vi "test Process Records.vi"(8 "error in":errorcluster, 11 "TestCase in":refnum<class "Engine.lvclass">) -> (0 "error out":errorcluster, 3 "TestCase out":refnum<class "Engine.lvclass">)   [LabVIEW 2020, in "Engine.lvclass"]
uses:
  Engine.lvclass
  Shared/RT Hardware Channel Settings.ctl
  Shared/RT Label Settings.ctl
  Shared/Label.ctl
  Shared/RT Parameters.ctl
  Shared/Parameter Definition.ctl
  <vilib>/NI/NI VeriStand Encoding and Decoding/Encoding.ctl
  <vilib>/NI VeriStand/Custom Device API/Custom Device Item Ref.ctl
  Shared/Transfer Type.ctl
  <vilib>/NI VeriStand/Custom Device API/Data Reference.ctl
  Shared/Map of Identifiers to Indexes.ctl
  <vilib>/addons/_JKI Toolkits/VI Tester/TestCase.llb/TestCase.lvclass
  <vilib>/NI VeriStand/Custom Device API/Custom Device API.lvlib
  <vilib>/NI/NI VeriStand Encoding and Decoding/Encoding and Decoding.lvlib
  Engine/Custom Device/Custom Device.lvlib
  Hardware API/AIM ARINC 429 Hardware API.lvlib
  C:/Program Files (x86)/National Instruments/LabVIEW 2020/vi.lib/addons/_JKI Toolkits/VI Tester/TestCase.llb/TestCase.lvclass
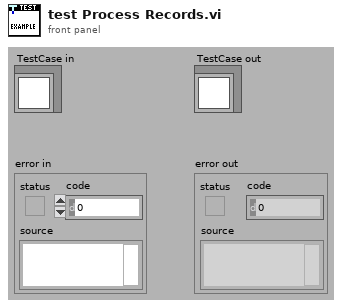
[diagram p1: front panel]
types:
  T1 = cluster{"type":u16, "count":u16, "timestamp":u32, "msgact":u16, "decgap":u16, "data":u32, "timestamph":u32}[]
  T2 = typedef "RT Hardware Channel Settings.ctl" = cluster{"channel #":u16, "channel handle":u64, "labels settings for RT":T3[]}
  T3 = typedef "RT Label Settings.ctl" = cluster{"Name":string, "xmlName":string, "label":T4, "transfer period":u32, "SDI_Enabled":bool, "SDI":u8, "parameter driver data":T5, "transfer type":T9, "has timestamp?":bool, "Label Disable/Trigger Channel Reference":T8, "Message Handle":u64, "Initialized?":bool, "Word Initial Raw Value":u32, "Label Timestamp Channel Data Reference":T10, "disabled":bool}
  T4 = typedef "Label.ctl" = u8
  T5 = typedef "RT Parameters.ctl" = cluster{"parameter definitions":T6[], "Tx parameter refs":T8[]}
  T6 = typedef "Parameter Definition.ctl" = cluster{"start index":i32, "size":i32, "encoding":T7, "signed":bool, "scale multiplier":dbl, "scale offset":dbl}
  T7 = typedef "Encoding and Decoding.lvlib/Encoding.ctl" = enum16{"BNR", "BCD", "Discrete"}
  T8 = typedef "Custom Device API.lvlib/Custom Device Item Ref.ctl" = u64
  T9 = typedef "Transfer Type.ctl" = enum16{"Scheduled", "Acyclic", "Block", "Strobe"}
  T10 = typedef "Custom Device API.lvlib/Data Reference.ctl" = i32
  T11 = typedef "Map of Identifiers to Indexes.ctl" = map{cluster{"Port":u8, "Label":u8, "SDI":u8}, cluster{"channel index":i32, "label index":i32, "start index":i32, "parameters":i32, "timestamp index":i32}}
  T12 = map{cluster{"hardware channel":u8, "label":u8, "SDI":u8}, cluster{"data word":u32, "time stamp":dbl}}
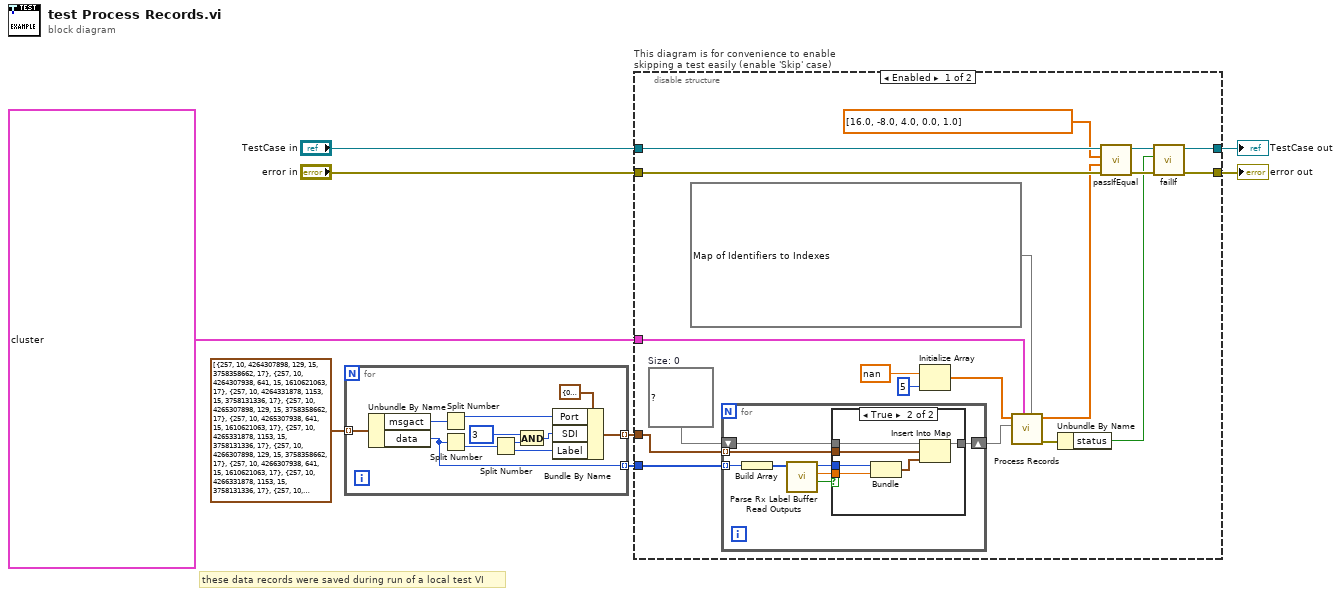
[diagram p0: block diagram]
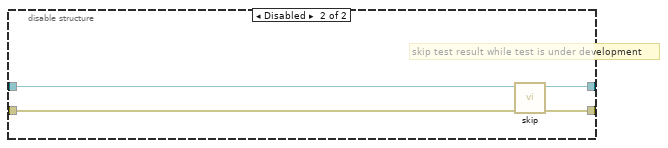
[diagram p3: hidden frame]
diagram:
  # "these data records were saved during run of a local test VI"
  n1 = for {
    tunnel: T1 [{"type"=257, "count"=10, "timestamp"=4264307898, "msgact"=129, "decgap"=15, "data"=3758358662, "timestamph"=17}, {"type"=257, "count"=10, "timestamp"=4264307938, "msgact"=641, "decgap"=15, "data"=1610621063, "timestamph"=17}, {"type"=257, "count"=10, "timestamp"=4264331878, "msgact"=1153, "decgap"=15, "data"=3758131336, "timestamph"=17}, {"type"=257, "count"=10, "timestamp"=4265307898, "msgact"=129, "decgap"=15, "data"=3758358662, "timestamph"=17}, {"type"=257, "count"=10, "timestamp"=4265307938, "msgact"=641, "decgap"=15, "data"=1610621063, "timestamph"=17}, {"type"=257, "count"=10, "timestamp"=4265331878, "msgact"=1153, "decgap"=15, "data"=3758131336, "timestamph"=17}, {"type"=257, "count"=10, "timestamp"=4266307898, "msgact"=129, "decgap"=15, "data"=3758358662, "timestamph"=17}, {"type"=257, "count"=10, "timestamp"=4266307938, "msgact"=641, "decgap"=15, "data"=1610621063, "timestamph"=17}, {"type"=257, "count"=10, "timestamp"=4266331878, "msgact"=1153, "decgap"=15, "data"=3758131336, "timestamph"=17}, {"type"=257, "count"=10, "timestamp"=4267307898, "msgact"=129, "decgap"=15, "data"=3758358662, "timestamph"=17}, {"type"=257, "count"=10, "timestamp"=4267307938, "msgact"=641, "decgap"=15, "data"=1610621063, "timestamph"=17}, {"type"=257, "count"=10, "timestamp"=4267331858, "msgact"=1153, "decgap"=15, "data"=3758131336, "timestamph"=17}, {"type"=257, "count"=10, "timestamp"=4268307898, "msgact"=129, "decgap"=15, "data"=3758358662, "timestamph"=17}, {"type"=257, "count"=10, "timestamp"=4268307938, "msgact"=641, "decgap"=15, "data"=1610621063, "timestamph"=17}, {"type"=257, "count"=10, "timestamp"=4268331858, "msgact"=1153, "decgap"=15, "data"=3758131336, "timestamph"=17}, {"type"=257, "count"=10, "timestamp"=4269307898, "msgact"=129, "decgap"=15, "data"=3758358662, "timestamph"=17}, {"type"=257, "count"=10, "timestamp"=4269307938, "msgact"=641, "decgap"=15, "data"=1610621063, "timestamph"=17}, {"type"=257, "count"=10, "timestamp"=4269331858, "msgact"=1153, "decgap"=15, "data"=3758131336, "timestamph"=17}, {"type"=257, "count"=10, "timestamp"=4270307898, "msgact"=129, "decgap"=15, "data"=3758358662, "timestamph"=17}, {"type"=257, "count"=10, "timestamp"=4270307938, "msgact"=641, "decgap"=15, "data"=1610621063, "timestamph"=17}, {"type"=257, "count"=10, "timestamp"=4270331878, "msgact"=1153, "decgap"=15, "data"=3758131336, "timestamph"=17}, {"type"=257, "count"=10, "timestamp"=4271307898, "msgact"=129, "decgap"=15, "data"=3758358662, "timestamph"=17}, {"type"=257, "count"=10, "timestamp"=4271307938, "msgact"=641, "decgap"=15, "data"=1610621063, "timestamph"=17}, {"type"=257, "count"=10, "timestamp"=4271331858, "msgact"=1153, "decgap"=15, "data"=3758131336, "timestamph"=17}, {"type"=257, "count"=10, "timestamp"=4272307898, "msgact"=129, "decgap"=15, "data"=3758358662, "timestamph"=17}, {"type"=257, "count"=10, "timestamp"=4272307938, "msgact"=641, "decgap"=15, "data"=1610621063, "timestamph"=17}, {"type"=257, "count"=10, "timestamp"=4272331858, "msgact"=1153, "decgap"=15, "data"=3758131336, "timestamph"=17}, {"type"=257, "count"=10, "timestamp"=4273307898, "msgact"=129, "decgap"=15, "data"=3758358662, "timestamph"=17}, {"type"=257, "count"=10, "timestamp"=4273307938, "msgact"=641, "decgap"=15, "data"=1610621063, "timestamph"=17}, {"type"=257, "count"=10, "timestamp"=4273331878, "msgact"=1153, "decgap"=15, "data"=3758131336, "timestamph"=17}, {"type"=257, "count"=10, "timestamp"=4274307898, "msgact"=129, "decgap"=15, "data"=3758358662, "timestamph"=17}, {"type"=257, "count"=10, "timestamp"=4274307938, "msgact"=641, "decgap"=15, "data"=1610621063, "timestamph"=17}, {"type"=257, "count"=10, "timestamp"=4274331858, "msgact"=1153, "decgap"=15, "data"=3758131336, "timestamph"=17}, {"type"=257, "count"=10, "timestamp"=4275307898, "msgact"=129, "decgap"=15, "data"=3758358662, "timestamph"=17}, {"type"=257, "count"=10, "timestamp"=4275307938, "msgact"=641, "decgap"=15, "data"=1610621063, "timestamph"=17}, {"type"=257, "count"=10, "timestamp"=4275331858, "msgact"=1153, "decgap"=15, "data"=3758131336, "timestamph"=17}, {"type"=257, "count"=10, "timestamp"=4276307898, "msgact"=129, "decgap"=15, "data"=3758358662, "timestamph"=17}, {"type"=257, "count"=10, "timestamp"=4276307938, "msgact"=641, "decgap"=15, "data"=1610621063, "timestamph"=17}, {"type"=257, "count"=10, "timestamp"=4276331858, "msgact"=1153, "decgap"=15, "data"=3758131336, "timestamph"=17}, {"type"=257, "count"=10, "timestamp"=4277307898, "msgact"=129, "decgap"=15, "data"=3758358662, "timestamph"=17}, {"type"=257, "count"=10, "timestamp"=4277307938, "msgact"=641, "decgap"=15, "data"=1610621063, "timestamph"=17}, {"type"=257, "count"=10, "timestamp"=4277331858, "msgact"=1153, "decgap"=15, "data"=3758131336, "timestamph"=17}] ("records") -> [w19] mode=indexing
    tunnel: [w12] -> w2 mode=indexing
    tunnel: [w9] -> w1 mode=indexing
    n2 = Unbundle By Name(w19) -> ("msgact"=w18:u16, "data"=w12:u32)
    n3 = Split Number(x=w18) -> (hi(x)=w16:u8)  [unwired: 1 out]
    n4 = Split Number(x=w12) -> (lo(x)=w13:u16)  [unwired: 1 out]
    n5 = Split Number(x=w13) -> (hi(x)=w14:u8, lo(x)=w10:u8)
    n6 = And(x=u8 3, y=w14) -> (x .and. y?=w11:u8)
    n7 = Bundle By Name(cluster=cluster{"Port":u8, "Label":u8, "SDI":u8} {"Port"=0, "Label"=134, "SDI"=0} ("message info"), "Port"=w16, "SDI"=w11, "Label"=w10) -> (w9:cluster{"Port":u8, "Label":u8, "SDI":u8})
  }
  n8 = disable-structure "This diagram is for convenience to enable skipping a test easily (enable 'Skip' case)" shown="Enabled" {
    disable-tunnel: "TestCase in" -> [w34 w57]
    disable-tunnel: [w38 w55] -> w5
    disable-tunnel: [w37 w56] -> w7
    disable-tunnel: "error in" -> [w33 w54]
    disable-tunnel: T2[] data[160728B] ("RT hardware channel data") -> [w24 _]
    disable-tunnel: w2 -> [w21 _]
    disable-tunnel: w1 -> [w20 _]
    frame Enabled {
      w23 = T12 {}  # Size: 0
      n9 = for {
        shift-right: [w44] -> w22
        shift-left: w23 -> [w45]
        tunnel: w21 -> [w41] mode=indexing
        tunnel: w20 -> [w39] mode=indexing
        n10 = Build Array(w41) -> (w40:u32[])
        n11 = call "Parse Rx Label Buffer Read Outputs.vi"("px_LData"=w40) -> ("hit"=w42:bool, "time stamp"=w46:dbl, "data word"=w43:u32)  [unwired: 6 in, 2 out]
        n12 = case shown="True" w42 {
          tunnel: w45 -> [w47 w52]
          tunnel: [w47 w53] -> w44
          tunnel: w39 -> [_ w51]
          tunnel: w43 -> [_ w50]
          tunnel: w46 -> [_ w48]
          frame False {
          }
          frame True {
            n13 = Bundle("data word"=w50, "time stamp"=w48) -> (w49:cluster{"data word":u32, "time stamp":dbl})  [unwired: 1 in]
            n14 = Insert Into Map(map in=w52, key=w51, value=w49) -> (map out=w53:T12)  [unwired: 2 out]
          }
        }
      }
      n15 = Initialize Array(nan ("element"), 5 ("dimension size")) -> (w27:dbl[])
      n16 = call "Process Records.vi"("map from message info to indexes"=T11 {{"Port"=0, "Label"=134, "SDI"=0}={"channel index"=0, "label index"=134, "start index"=0, "parameters"=1, "timestamp index"=-1}, {"Port"=2, "Label"=135, "SDI"=0}={"channel index"=2, "label index"=135, "start index"=1, "parameters"=1, "timestamp index"=-1}, {"Port"=4, "Label"=136, "SDI"=0}={"channel index"=4, "label index"=136, "start index"=2, "parameters"=3, "timestamp index"=-1}} ("map"), "RT hardware channel data"=w24, "map from message info to data word"=w22, "parameter values in"=w27) -> ("error out"=w32:errorcluster, "parameter values out"=w26:dbl[])  [unwired: 4 in]
      n17 = Unbundle By Name(w32) -> ("status"=w31:bool)
      n18 = call-dynamic "passIfEqual.vi"("error in (no error)"=w33, "y"=w26, "x"=dbl[] [16.0, -8.0, 4.0, 0.0, 1.0] ("parameter values out"), "TestCase in"=w34) -> ("error out"=w35:errorcluster, "TestCase out"=w36:refnum<class "Engine.lvclass">)  [unwired: 6 in]
      n19 = call-dynamic "failIf.vi"("error in (no error)"=w35, "fail"=w31, "TestCase in"=w36) -> ("error out"=w37:errorcluster, "TestCase out"=w38:refnum<class "Engine.lvclass">)  [unwired: 7 in]
    }
    frame Disabled {
      # "skip test result while test is under development"
      n20 = call <vilib>:"skip.vi"("error in (no error)"=w54, "TestCase in"=w57) -> ("error out"=w56:errorcluster, "TestCase out"=w55:refnum<class "Engine.lvclass">)  [unwired: 8 in]
    }
  }
  "error out" <- w7
  "TestCase out" <- w5
